vi "Draw Tree.vi"(8 "error in":errorcluster, 10 "Tree Control Items":T1(array[cluster]), 11 "TreeControl in":refnum<vi>) -> (0 "error out":errorcluster)   [LabVIEW 2020, in "Panter Dashboard.lvlib"]
uses:
  Panter Dashboard.lvlib
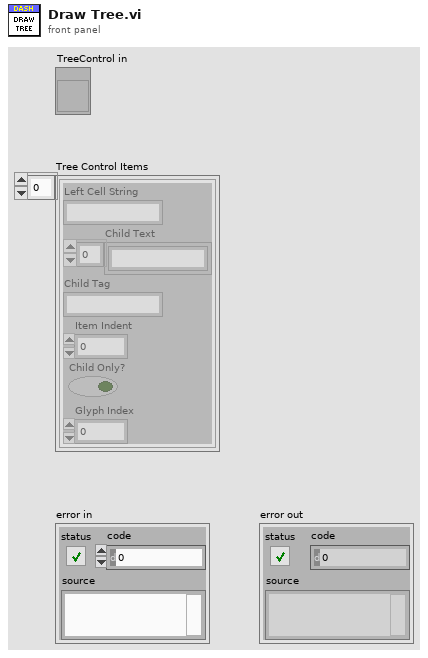
[diagram p1: front panel]
types:
  T1 = cluster{"Left Cell String":string, "Child Text":string[], "Child Tag":string, "Item Indent":i32, "Child Only?":bool, "Glyph Index":i32}[]
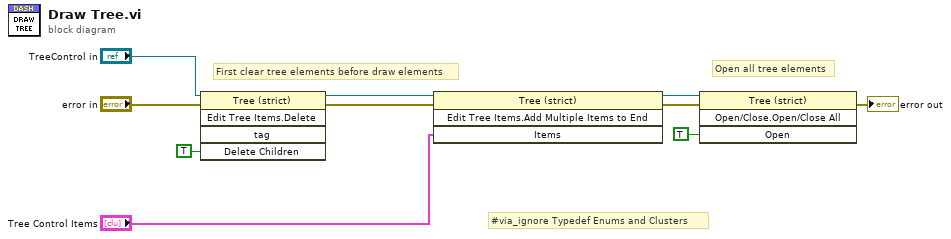
[diagram p0: block diagram]
diagram:
  # "Open all tree elements"
  # "First clear tree elements before draw elements"
  # "#via_ignore Typedef Enums and Clusters"
  n1 = invoke class="Tree (strict)" method="Edit Tree Items.Delete"(reference="TreeControl in", error in="error in", "Delete Children"=TRUE ("Delete Children?")) -> (reference out=w2:refnum<vi>, error out=w7:errorcluster)  [unwired: 2 in, 3 out]
  n2 = invoke on="Invoke Node" class="Tree (strict)" method="Edit Tree Items.Add Multiple Items to End"(reference=w2, error in=w7, "Items"="Tree Control Items") -> (reference out=w5:refnum<vi>, error out=w10:errorcluster)  [unwired: 1 in, 2 out]
  n3 = invoke class="Tree (strict)" method="Open/Close.Open/Close All"(reference=w5, error in=w10, "Open"=TRUE ("Open?")) -> (error out=→"error out":errorcluster)  [unwired: 1 in, 3 out]
